vi "Synthesize.vi"(0 "Pulse Train in":refnum<class "Pulse Train.lvclass">, 5 "Fs (Hz)":dbl, 7 "Npts":i32, 9 "Repetition":i32, 11 "error in (no error)":errorcluster) -> (4 "Pulse Train out":refnum<class "Pulse Train.lvclass">, 8 "Array":dbl[](array[numeric]), 15 "error out":errorcluster)   [LabVIEW 2020, in "Pulse Train.lvclass"]
uses:
  Pulse Train.lvclass
  Pulse Train.lvclass/Pulse Train.ctl
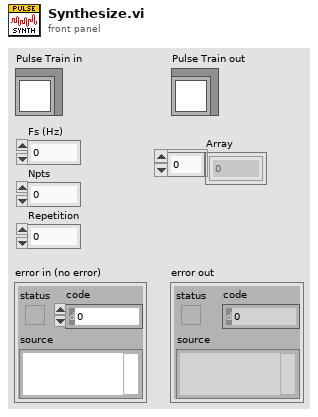
[diagram p1: front panel]
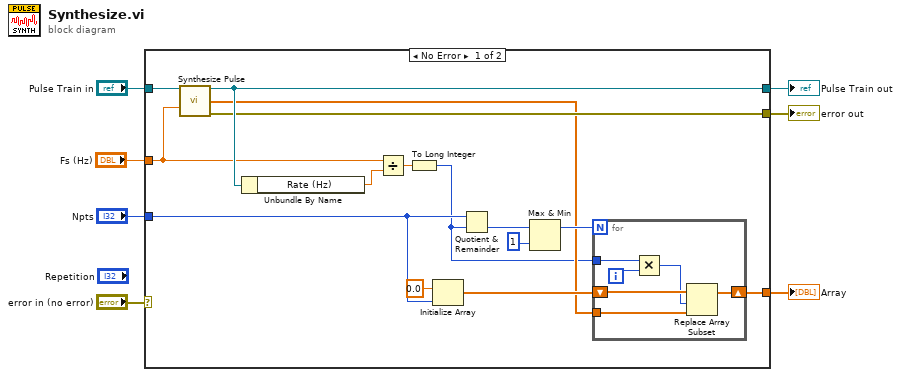
[diagram p0: block diagram]
diagram:
  n1 = case shown="No Error" "error in (no error)" {
    tunnel: "Pulse Train in" -> [w22 w29]
    tunnel: [w15 w29] -> w5
    tunnel: "Fs (Hz)" -> [w13 _]
    tunnel: "Npts" -> [w12 _]
    tunnel: [w11 _] -> w2
    tunnel: [w10 _] -> w1
    frame No Error {
      n2 = call "Synthesize Pulse.vi"("Pulse Train in"=w22, "Fs (Hz)"=w13) -> ("Pulse Train out"=w15:refnum<class "Pulse Train.lvclass">, "Pulse"=w9:dbl[], "error out"=w11:errorcluster)  [unwired: 11 in]
      n3 = Unbundle By Name(w15) -> ("Rate (Hz)"=w14:dbl)
      n4 = Divide(x=w13, y=w14) -> (x/y=w16:dbl)
      n5 = To Long Integer(number=w16) -> (32bit integer=w8:i32)
      n6 = Initialize Array(0.0 ("element"), w12) -> (w18:dbl[])
      n7 = Quotient & Remainder(x=w12, y=w8) -> (floor(x/y)=w20:i32)  [unwired: 1 out]
      n8 = Max & Min(x=w20, y=1 ("x")) -> (max(x,y)=w19:i32)  [unwired: 1 out]
      n9 = for {
        N: w19 -> [_]
        tunnel: w9 -> [w26]
        shift-right: [w27] -> w10
        shift-left: w18 -> [w28]
        tunnel: w8 -> [w25]
        i -> [w24]
        n10 = Multiply(x=w25, y=w24) -> (x*y=w23:i32)
        n11 = Replace Array Subset(array=w28, new element=w26, index=w23) -> (w27:dbl[])
      }
    }
    frame Error {
    }
  }
  "error out" <- w2
  "Pulse Train out" <- w5
  "Array" <- w1
